vi "Add 5 Task.vi"(11 "Promise":refnum<class "Promise.lvclass">) -> ()   [LabVIEW 2020, in "Futures-Examples.lvlib"]
uses:
  Futures-Examples.lvlib
  Promises/Promise/Promise.lvclass
  DoubleValue/DoubleValue.lvclass
  C:/dev/lv/2020/lv-promises/Promises/Value/Value.lvclass
  DoubleValue/DoubleValue.lvclass/DoubleValue.ctl
  1c47de9d-079d-40aa-9345-8a96c69ffcdd.vi
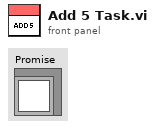
[diagram p1: front panel]
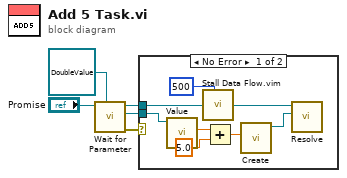
[diagram p0: block diagram]
diagram:
  n1 = call "Wait for Parameter.vi"("Param Type (Default)"=refnum<class "DoubleValue.lvclass"> refnum ("Futures-Examples.lvlib:DoubleValue.lvclass"), "Promise in"="Promise") -> ("error out"=w1:errorcluster, "Parameter"=w3:refnum<class "DoubleValue.lvclass">, "Promise out"=w2:refnum<class "Promise.lvclass">)  [unwired: 7 in]
  n2 = case shown="No Error" w1 {
    tunnel: w3 -> [w13 _]
    tunnel: w2 -> [w9 _]
    frame No Error {
      n3 = call "Value.vi"("DoubleValue in"=w13) -> ("Value"=w12:dbl)  [unwired: 10 in]
      n4 = call "Stall Data Flow.vim"("value in"=w9, "milliseconds to wait"=u32 500) -> ("value out"=w7:refnum<class "Promise.lvclass">)  [unwired: 1 out]
      n5 = Add(x=w12, y=5.0) -> (x+y=w10:dbl)
      n6 = call "Create.vi"("Value"=w10) -> ("DoubleValue"=w8:refnum<class "DoubleValue.lvclass">)  [unwired: 10 in]
      n7 = call "Resolve.vi"("Result"=w8, "Promise in"=w7) -> ()  [unwired: 8 in, 2 out]
    }
    frame Error {
    }
  }
